vi "filtr_b.vi"(7 "count?":bool, 8 "threshold":i32=1, 11 "input array":dbl[][](array[numeric])) -> (3 "output array":dbl[][](array[numeric]))   [LabVIEW 2017]
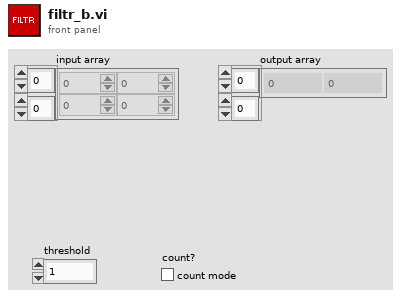
[diagram p1: front panel]
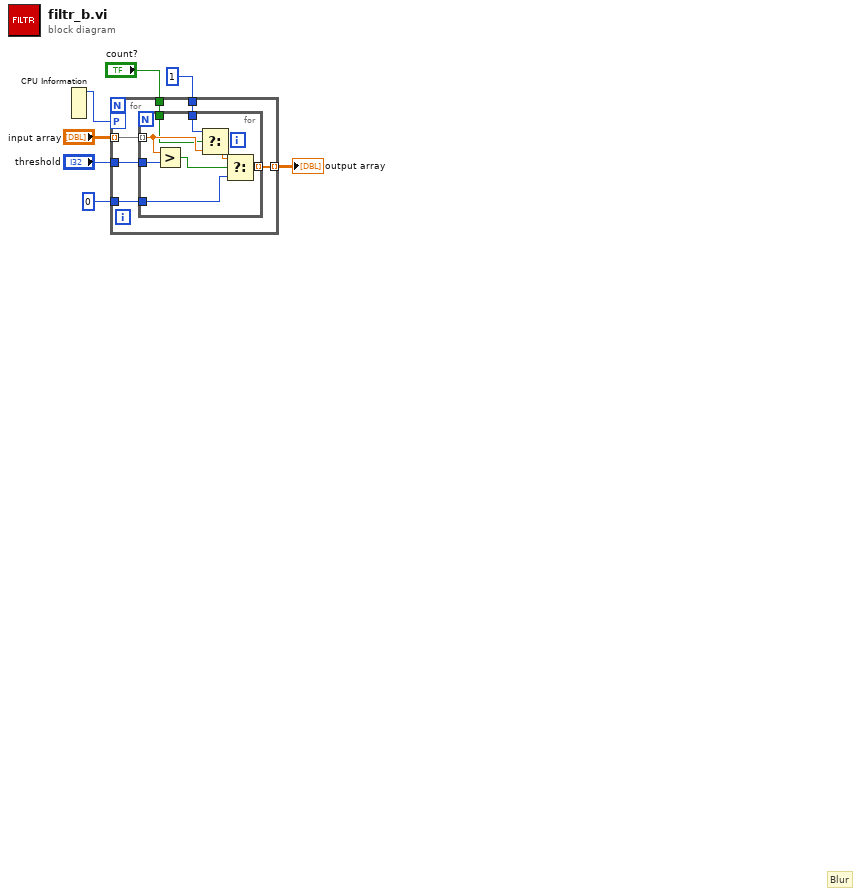
[diagram p0: block diagram]
diagram:
  # "Blur"
  n1 = CPU Information() -> (4:w3:i32)  [unwired: 3 out]
  n2 = for {
    tunnel: "input array" -> [w13] mode=indexing
    tunnel: "threshold" -> [w12]
    tunnel: [w11] -> w5 mode=indexing
    workers-P: w3 -> [_]
    tunnel: 0 -> [w10]
    tunnel: 1 -> [w9]
    tunnel: "count?" -> [w8]
    n3 = for {
      tunnel: w13 -> [w17] mode=indexing
      tunnel: w12 -> [w19]
      tunnel: [w20] -> w11 mode=indexing
      tunnel: w10 -> [w21]
      tunnel: w9 -> [w16]
      tunnel: w8 -> [w15]
      n4 = Greater?(x=w17, y=w19) -> (0:w18:bool)
      n5 = Select(t=w16, s=w15, f=w17) -> (s? t:f=w14:dbl)
      n6 = Select(t=w14, s=w18, f=w21) -> (s? t:f=w20:dbl)
    }
  }
  "output array" <- w5
